vi "Memory Management.MoveByteBlock.Write (String).vi"(0 "src ptr in":u64, 1 "src offset (0)":u64, 2 "dst in":string, 3 "dst offset (0)":u64, 4 "size":u64, 5 "error in (no error)":errorcluster) -> (14 "src ptr out":u64, 15 "src offset out":u64, 16 "dst out":string, 17 "dst offset out":u64, 18 "size out":u64, 19 "error out":errorcluster)   [LabVIEW 2016, in "VeriStand Data.lvlib"]
doc: "Calls into VeriStand's Data Services library to move a data block of length <B>size</B> from the <B>src</B> to <B>dst</B>."
uses:
  VeriStand Data.lvlib
  <vilib>/NI Veristand/Custom Device API/data/NIVeriStand_DataServices.dll
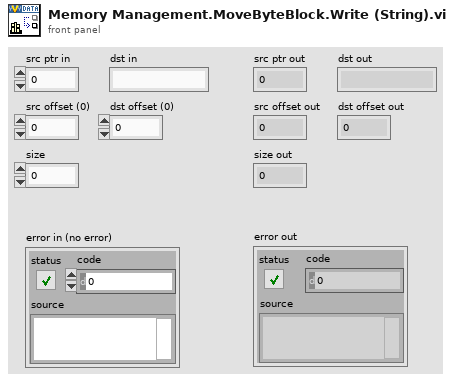
[diagram p1: front panel]
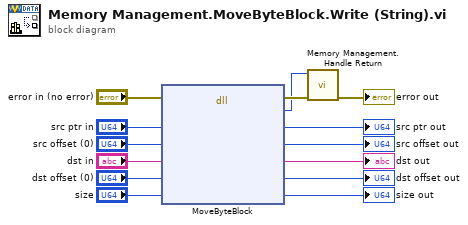
[diagram p0: block diagram]
diagram:
  n1 = dll-call lib="C:/Program Files (x86)/National Instruments/LabVIEW 2016/vi.lib/NI Veristand/Custom Device API/data/NIVeriStand_DataServices.*" fn="MoveByteBlock"(error in="error in (no error)", "srcPtr"="src ptr in", "srcOffset"="src offset (0)", "dstPtr"="dst in", "dstOffset"="dst offset (0)", "count"="size") -> (error out=w6:errorcluster, "return type"=w4:i32, "srcPtr"=→"src ptr out":u64, "srcOffset"=→"src offset out":u64, "dstPtr"=→"dst out":string, "dstOffset"=→"dst offset out":u64, "count"=→"size out":u64)  [unwired: 2 in, 1 out]
  n2 = call "Memory Management.Handle Return.vi"("error in (no error)"=w6, "return"=w4) -> ("error out"=→"error out":errorcluster)  [unwired: 9 in]
